vi "Experiment header-initialise.vi"(8 "error in (no error)":errorcluster, 10 "AOL_Globals":T1={"Imaging Protocol"=enum."AOL Z-Stack", "Number of POI"=0, "Number of Miniscans"=0, "Number of Trials"=0, "Number of Cycles "=0, "# Averaged Frames"=0, "Laser power (%)"=0, "Pockels (V)"=0.0, "Acquisition Length (sec)"=0.0, "Fill time (us)"=0.0, "POI Dwell time (us)"=0.0, "Miniscan Dwell time per pixel (us)"=0.0, "PMT 1"=0.0, "PMT 2"=0.0, "Back Apperture (mA)"=200.0, "Frame Size"=0, "Center Frequency"=0.0, "Field of View (norm)"=0.0, "DwellTime (us)"=0.0, "Wavelength (nm)"=0.0, "Zoom"=0.0, "AOL Z"=0.0, "AOL Mode"=enum."Raster", "GridXY"=0.0, "GridZ"=0.0, "TriggerPeriod (sec)"=0.0, "Number of Pixels in Miniscan"=0, "Experiment folder path"=path "", "X centre"=0.0, "Y centre"=0.0, "Angle (degrees)"=0.0, "Plane Mode"=0, "Threshold"=[], "Regenerate Chirps"=FALSE, "Rectangle ROI length (pixels)"=0, "Rectangle ROI height (pixels)"=0, "AOD fill"=4900, "StartupDelay"=0, "Samples Wait after Trigger"=5080, "Slip Cycle"=600000, "Add Cycle"=TRUE, "Functional Mode"=enum."Point", "Z Start"=0.0, "Z Stop"=0.0, "# Planes"=0} {"Plane Mode" items=["XY Plane", "XZ Plane", "YZ Plane", "arbitraryplane"]; "Frame Size" items=["100X100"=100, "128X128"=128, "200X200"=200, "256X256"=256, "512X512"=512, "1024x1024"=1024, "2048x2048"=2048]; "Back Apperture (mA)" format="%#.6g"; "Pockels (V)" format="%#.6g"; "PMT 2" format="%#.6g"; "PMT 1" format="%#.6g"; "Angle (degrees)" format="%#.6g"; "POI Dwell time (us)" format="%#.6g"}, 11 "Experiment data folder path":path) -> (0 "error out":errorcluster)   [LabVIEW 2017]
uses:
  Typedefs/Controls/AOL_Globals.ctl
  Typedefs/Imaging Protocols enum.ctl
  Typedefs/Frame Size.ctl
  Typedefs/AOL modes.ctl
  Typedefs/Plane Mode.ctl
  Typedefs/Functional Mode.ctl
  Typedefs/Header file sections.ctl
  Typedefs/Header file interface module functions enum.ctl
panel:
  # "<------Place holder only - not in use"
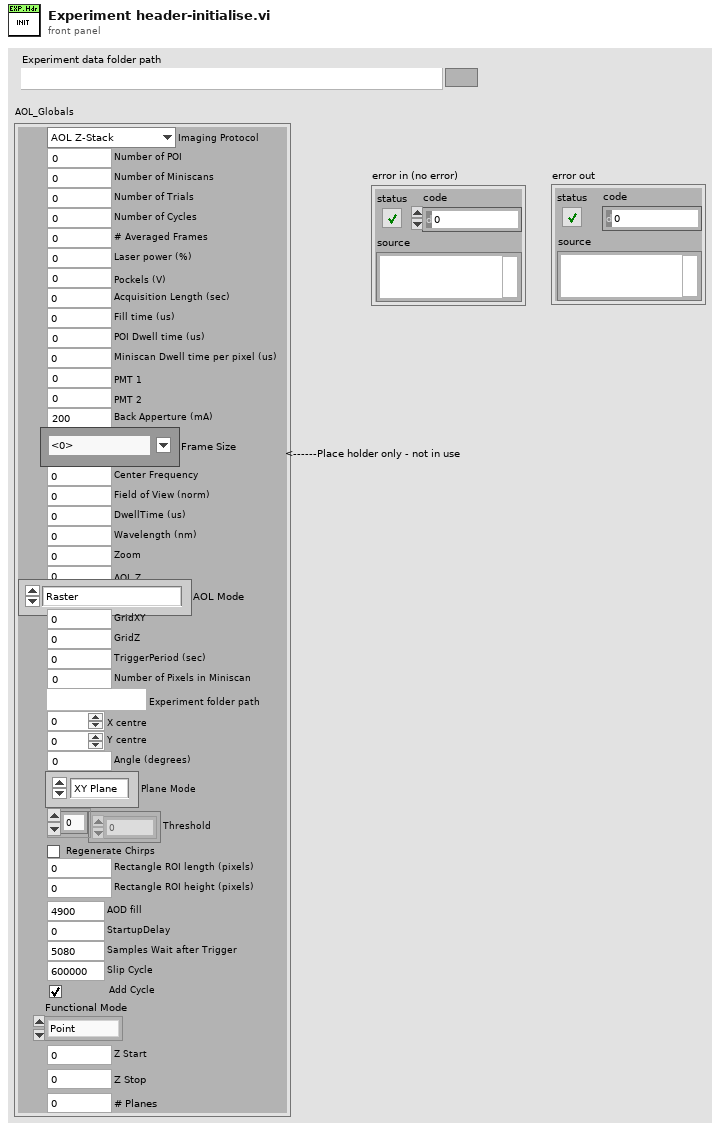
[diagram p1: front panel]
types:
  T1 = typedef "AOL_Globals.ctl" = cluster{"Imaging Protocol":T2, "Number of POI":u16, "Number of Miniscans":u16, "Number of Trials":u16, "Number of Cycles ":u64, "# Averaged Frames":u16, "Laser power (%)":u8, "Pockels (V)":dbl, "Acquisition Length (sec)":dbl, "Fill time (us)":dbl, "POI Dwell time (us)":dbl, "Miniscan Dwell time per pixel (us)":dbl, "PMT 1":dbl, "PMT 2":dbl, "Back Apperture (mA)":dbl, "Frame Size":T3, "Center Frequency":dbl, "Field of View (norm)":dbl, "DwellTime (us)":dbl, "Wavelength (nm)":dbl, "Zoom":dbl, "AOL Z":dbl, "AOL Mode":T4, "GridXY":dbl, "GridZ":dbl, "TriggerPeriod (sec)":dbl, "Number of Pixels in Miniscan":u16, "Experiment folder path":path, "X centre":dbl, "Y centre":dbl, "Angle (degrees)":dbl, "Plane Mode":T5, "Threshold":u16[], "Regenerate Chirps":bool, "Rectangle ROI length (pixels)":u16, "Rectangle ROI height (pixels)":u16, "AOD fill":u16, "StartupDelay":i32, "Samples Wait after Trigger":u16, "Slip Cycle":u32, "Add Cycle":bool, "Functional Mode":T6, "Z Start":dbl, "Z Stop":dbl, "# Planes":i32}
  T2 = typedef "Imaging Protocols enum.ctl" = enum16{"AOL Z-Stack", "Motor Z Stack", "Functional Acquisition", "Single Plane Acquisition", "Volume Acquisition", "Live Imaging", "Live Plane Imaging", "Live Volume Imaging"}
  T3 = typedef "Frame Size.ctl" = u16
  T4 = typedef "AOL modes.ctl" = enum16{"Raster", "Structural", "Pointing", "Mini Scan", "Alignment"}
  T5 = typedef "Plane Mode.ctl" = u16
  T6 = typedef "Functional Mode.ctl" = enum16{"Point", "Line", "Patch", "Plane", "Volume"}
  T7 = typedef "Header file interface module functions enum.ctl" = enum16{"Load experiment header file", "Save experiment header file", "Clear stored values", "Read stored values", "Update specific value in memory", "Update values in memory"}
  T8 = typedef "Header file sections.ctl" = enum16{"ALL SECTIONS", "LOGIN", "GLOBAL PARAMETERS", "IMAGING MODES", "TIME SERIES", "MOTOR Z-STACK", "AOL Z-STACK", "FUNCTIONAL IMAGING", "VOLUME IMAGING", "MOVEMENT CORRECTION", "CALIBRATION", "STATISTICS", "BIOLOGY INFORMATION"}
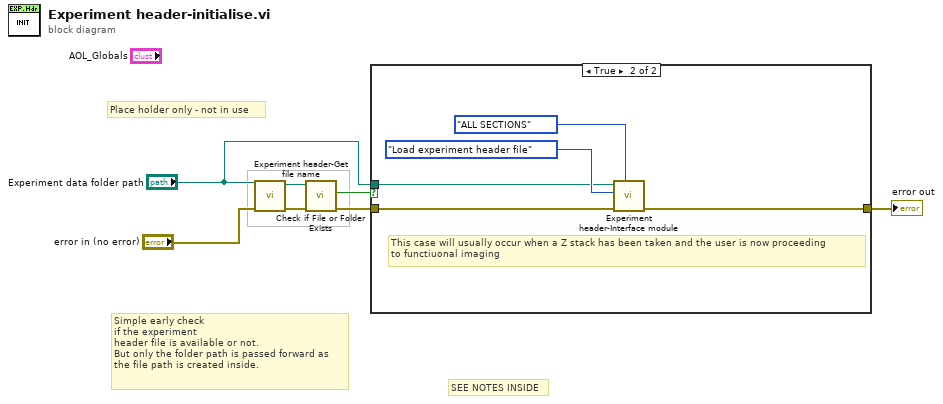
[diagram p0: block diagram]
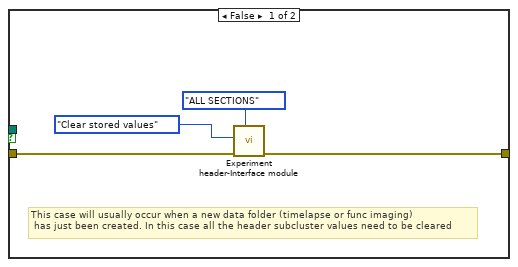
[diagram p2: hidden frame]
diagram:
  # "Simple early check\nif the experiment\nheader file is available or not.\nBut only the folder path is passed forward as\nthe file path is created inside."
  # "Place holder only - not in use"
  # "SEE NOTES INSIDE"
  n1 = call "Experiment header-Get file name.vi"("error in (no error)"="error in (no error)", "Experiment data folder path"="Experiment data folder path") -> ("error out"=w5:errorcluster, "Header File Path"=w6:path)  [unwired: 8 in]
  n2 = call <vilib>:"Check if File or Folder Exists.vi"("error in (no error)"=w5, "path"=w6) -> ("error out"=w3:errorcluster, "file or folder exists?"=w4:bool)  [unwired: 7 in, 1 out]
  n3 = case shown="True" w4 {
    tunnel: w3 -> [w11 w14]
    tunnel: "Experiment data folder path" -> [_ w13]
    tunnel: [w8 w12] -> w2
    frame False {
      # "This case will usually occur when a new data folder (timelapse or func imaging)\n has just been created. In this case all the header subcluster values need to be cleared"
      n4 = call "Experiment header-Interface module.vi"("Header file sections"=Header_file_sections."ALL SECTIONS", "error in (no error)"=w11, "Function"=Header_file_interface_module_functions_enum."Clear stored values") -> ("error out"=w8:errorcluster)  [unwired: 7 in, 1 out]
    }
    frame True {
      # "This case will usually occur when a Z stack has been taken and the user is now proceeding\nto functiuonal imaging"
      n5 = call "Experiment header-Interface module.vi"("Header file sections"=Header_file_sections."ALL SECTIONS", "error in (no error)"=w14, "Function"=Header_file_interface_module_functions_enum."Load experiment header file", "Experiment data folder path"=w13) -> ("error out"=w12:errorcluster)  [unwired: 6 in, 1 out]
    }
  }
  "error out" <- w2
